vi "通信.vi"(8 "error in (no error)":errorcluster, 10 "Slave ID":u8=1, 11 "MB session in":refnum<class "MB_Master.lvclass">) -> (0 "error out":errorcluster, 2 "读取值":T1, 3 "MB session out":refnum<class "MB_Master.lvclass">)   [LabVIEW 2016, in "流量计集成.lvlib" / "LSS-100X流量计.lvlib"]
uses:
  <vilib>/Plasmionique/MB Master/MB_Master/MB_Master.lvclass
  <vilib>/Plasmionique/MB Master/MB Master.lvlib
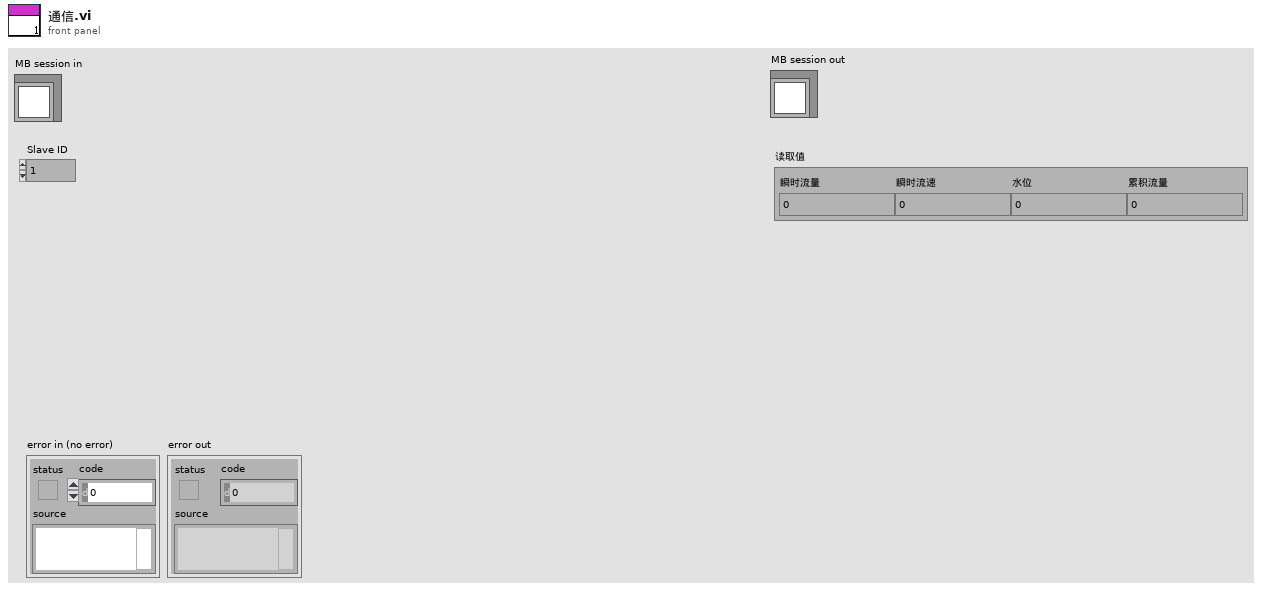
[diagram p1: front panel]
types:
  T1 = typedef "流量计集成.lvlib/LSS-100X流量计.lvlib/读取值.ctl" = cluster{"瞬时流量":sgl, "瞬时流速":sgl, "水位":sgl, "累积流量":i32}
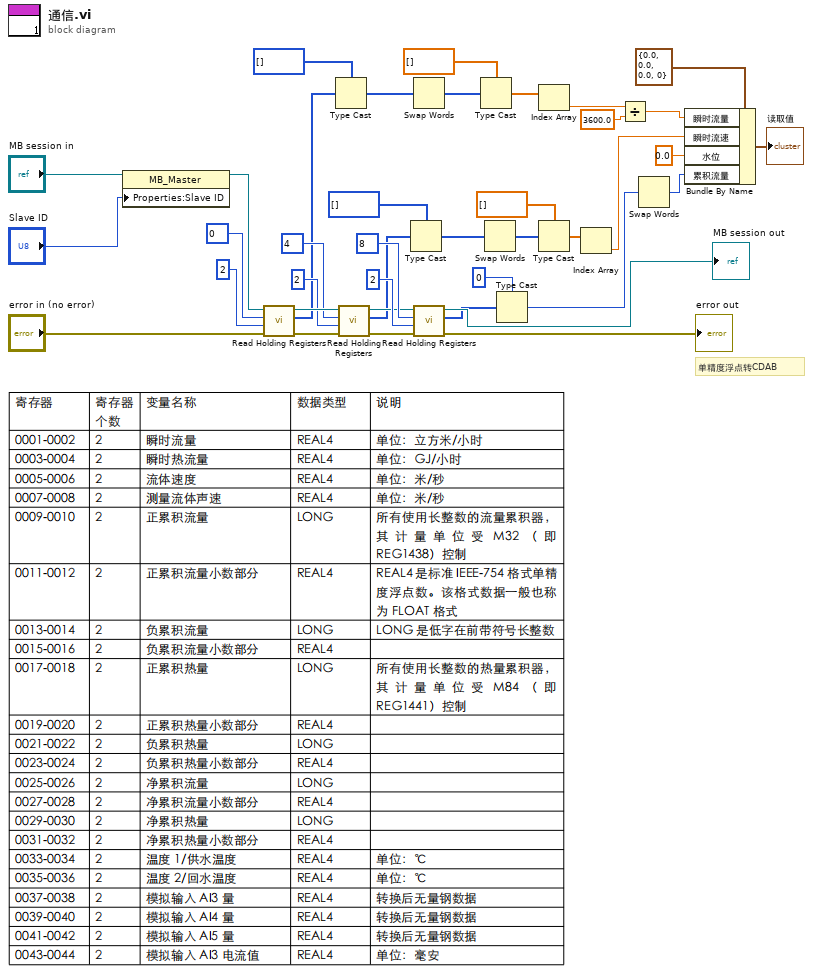
[diagram p0: block diagram]
diagram:
  # "单精度浮点转CDAB"
  n1 = property class="MB_Master"(reference="MB session in", "Properties:Slave ID"="Slave ID") -> (reference out=w33:refnum<class "MB_Master.lvclass">)  [unwired: 1 in, 1 out]
  n2 = call <vilib>:"Read Holding Registers.vi"("error in (no error)"="error in (no error)", "quantity"=u16 2, "starting address"=u16 0, "MB session in"=w33) -> ("error out"=w37:errorcluster, "Registers"=w14:u16[], "MB session out"=w38:refnum<class "MB_Master.lvclass">)  [unwired: 5 in]
  n3 = Type Cast(type=u32[] [], x=w14) -> (*(type *) &x=w16:u32[])
  n4 = call <vilib>:"Read Holding Registers.vi"("error in (no error)"=w37, "quantity"=u16 2, "starting address"=u16 4, "MB session in"=w38) -> ("error out"=w22:errorcluster, "Registers"=w7:u16[], "MB session out"=w23:refnum<class "MB_Master.lvclass">)  [unwired: 5 in]
  n5 = Type Cast(type=u32[] [], x=w7) -> (*(type *) &x=w10:u32[])
  n6 = Swap Words(1:w16) -> (0:w15:u32[])
  n7 = call <vilib>:"Read Holding Registers.vi"("error in (no error)"=w22, "quantity"=u16 2, "starting address"=u16 8, "MB session in"=w23) -> ("error out"=→"error out":errorcluster, "Registers"=w24:u16[], "MB session out"=→"MB session out":refnum<class "MB_Master.lvclass">)  [unwired: 5 in]
  n8 = Type Cast(type=sgl[] [], x=w15) -> (*(type *) &x=w13:sgl[])
  n9 = Swap Words(1:w10) -> (0:w11:u32[])
  n10 = Type Cast(type=0 ("x/y"), x=w24) -> (*(type *) &x=w2:i32)
  n11 = Index Array(array=w13) -> (element=w5:sgl)  [unwired: 1 in]
  n12 = Type Cast(type=sgl[] [], x=w11) -> (*(type *) &x=w12:sgl[])
  n13 = Index Array(array=w12) -> (element=w6:sgl)  [unwired: 1 in]
  n14 = Divide(x=w5, y=sgl 3600.0) -> (x/y=w3:sgl)
  n15 = Swap Words(1:w2) -> (0:w1:i32)
  n16 = Bundle By Name(cluster=T1 {"瞬时流量"=0.0, "瞬时流速"=0.0, "水位"=0.0, "累积流量"=0} ("读取值"), "瞬时流量"=w3, "瞬时流速"=w6, "水位"=sgl 0.0 ("x/y"), "累积流量"=w1) -> (→"读取值":T1)
